vi "set gamma.vi"(8 "error in (no error)":errorcluster, 11 "Thorcam in":refnum<class "Thorcam.lvclass">) -> (0 "error out":errorcluster, 3 "Thorcam out":refnum<class "Thorcam.lvclass">)   [LabVIEW 2012, in "Thorcam.lvclass"]
uses:
  Thorcam.lvclass
  Thorcam.lvclass/Thorcam.ctl
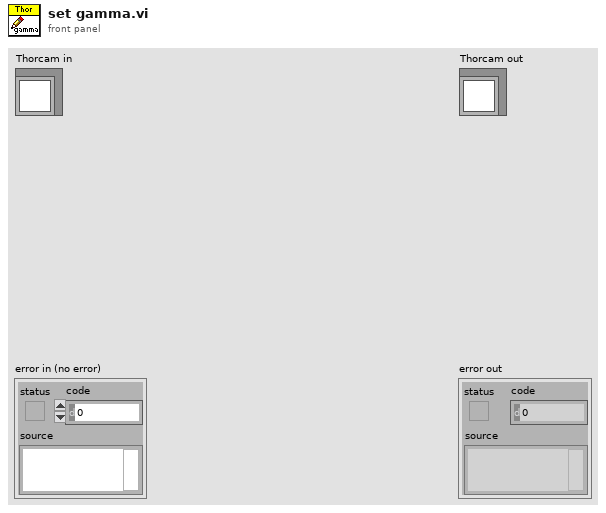
[diagram p1: front panel]
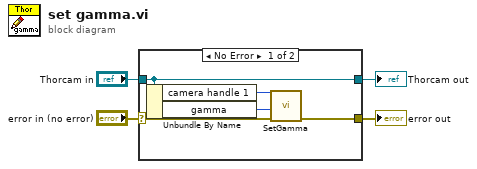
[diagram p0: block diagram]
diagram:
  n1 = case shown="No Error" "error in (no error)" {
    selector: "error in (no error)" -> [w7 w11]
    tunnel: [w6 w11] -> w3
    tunnel: [w9 w10] -> w1
    tunnel: "Thorcam in" -> [w9 w10]
    frame No Error {
      n2 = Unbundle By Name(w9) -> ("camera handle 1"=w8:u32, "gamma"=w5:i32)
      n3 = call <instrlib>:"SetGamma.vi"("error in"=w7, "Gamma"=w5, "Camera Handle In"=w8) -> ("error out"=w6:errorcluster)  [unwired: 7 in, 1 out]
    }
    frame Error {
    }
  }
  "error out" <- w3
  "Thorcam out" <- w1
